vi "Calibrate Camera.vi"(0 "Image In":T1, 5 "Image Dst":T1, 7 "File Path (Image Calibration 1)":path=path "C:/Users/wobot/OneDrive/Desktop/Calibrations/Dots/Cam2.png", 9 "Angle Relative to Horizontal (deg)":sgl, 11 "error in":errorcluster) -> (4 "Image Out":T1, 8 "Execution Time":u32, 15 "error out":errorcluster)   [LabVIEW 2025]
doc: "Creates, edits, and runs vision algorithms using NI Vision Assistant.\n\nWhen you place this Express VI on the block diagram, NI Vision Assistant launches. Create an algorithm using the Vision Assistant processing functions. After you create an algorithm, you can select the controls and indicators that you want to be able to programmatically set in LabVIEW. Double-click the Vision Assistant Express VI to edit the algorithm."
uses:
  <vilib>/vision/Image Controls.llb/IMAQ Image.ctl
  <vilib>/vision/NI_Vision_Development_Module.lvlib
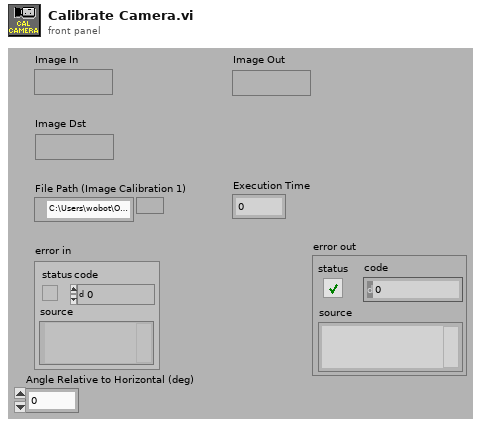
[diagram p1: front panel]
types:
  T1 = typedef "IMAQ Image.ctl" = refnum<image>
  T2 = cluster{"Origin Pixel":cluster{"X":sgl, "Y":sgl}, "Angle Relative to Horizontal (deg)":sgl, "Axis Reference":u32}
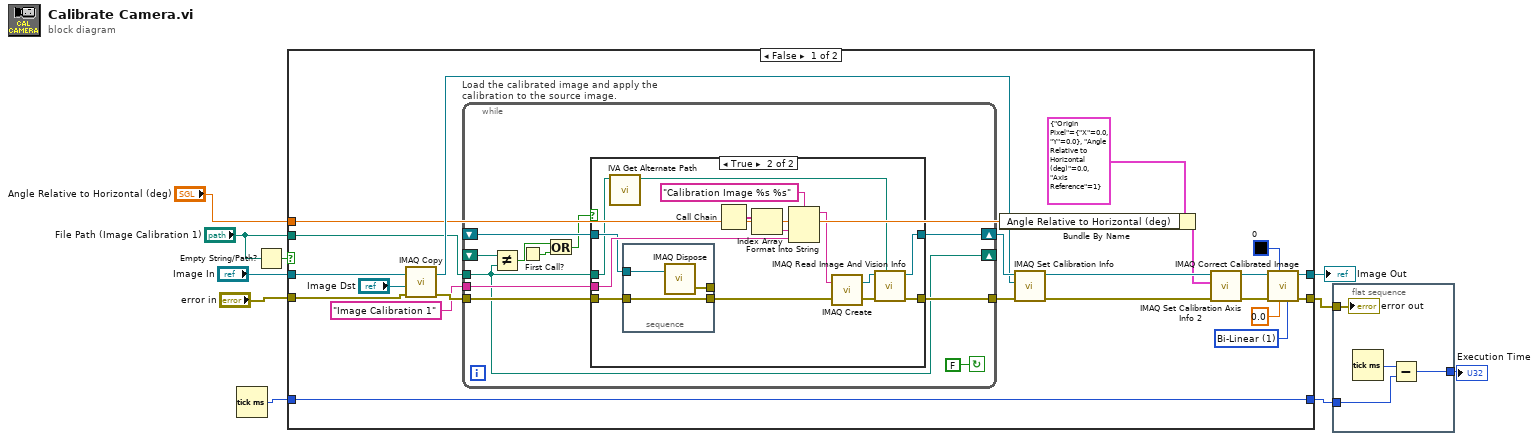
[diagram p0: block diagram]
diagram:
  n1 = Tick Count (ms)() -> (millisecond timer value=w5:u32)
  n2 = Empty String/Path?(string/path="File Path (Image Calibration 1)") -> (empty?=w7:bool)
  n3 = case shown="False" w7 {
    tunnel: "Image In" -> [w31 w64]
    tunnel: [w21 _] -> w4
    tunnel: [w17 w64] -> w9
    tunnel: "File Path (Image Calibration 1)" -> [w16 _]
    tunnel: "error in" -> [w15 _]
    tunnel: w5 -> [w14 w63]
    tunnel: [w14 w63] -> w3
    tunnel: "Angle Relative to Horizontal (deg)" -> [w11 _]
    frame False {
      w22 = u32 1 items=["Zero Order", "Bi-Linear", "Quadratic", "Cubic Spline"] ("Interpolation Type")
      n4 = call "IMAQ Copy"("error in (no error)"=w15, "Image Dst"="Image Dst", "Image Src"=w31) -> ("error out"=w30:errorcluster, "Image Dst Out"=w26:T1)  [unwired: 3 out]
      n5 = while "Load the calibrated image and apply the calibration to the source image." {
        shift-right: [w43] -> w29
        shift-left: _ -> [w42]
        tunnel: [w40] -> w28
        tunnel: w30 -> [w39]
        tunnel: w16 -> [w36]
        tunnel: "Image Calibration 1" ("Step Name") -> [w38]
        shift-right: [w36] -> _
        shift-left: _ -> [w37]
        stop <- FALSE continue-if-true
        n6 = Not Equal?(x=w37, y=w36) -> (x != y?=w34:bool)
        n7 = First Call?() -> (First Call?: T/F=w35:bool)
        n8 = Or(x=w34, y=w35) -> (x .or. y?=w33:bool)
        n9 = case shown="True" w33 {
          tunnel: [w45 w57] -> w43
          tunnel: w42 -> [w45 w49]
          tunnel: [w44 w54] -> w40
          tunnel: w39 -> [w44 w50]
          tunnel: w36 -> [_ w47]
          tunnel: w38 -> [_ w51]
          frame False {
          }
          frame True {
            n10 = call <vilib>:"IVA Get Alternate Path.vi"("Path In"=w47) -> ("Path Out"=w46:path)  [unwired: 10 out]
            n11 = stacked-sequence {
              tunnel: w50 -> [w61]
              tunnel: w49 -> [w62]
              tunnel: [w61] -> w48
              tunnel: [w60] -> _
              frame #0 {
                n12 = call "IMAQ Dispose"("Image"=w62) -> ("error out"=w60:errorcluster)  [unwired: 2 in, 3 out]
              }
            }
            n13 = Call Chain() -> (call chain=w53:string[])
            n14 = Index Array(array=w53) -> (element=w52:string)  [unwired: 1 in]
            n15 = Format Into String(format string="Calibration Image %s %s" ("Image Name"), w52, w51) -> (resulting string=w59:string)  [unwired: 2 in, 1 out]
            n16 = call "IMAQ Create"("Image Name"=w59, "error in (no error)"=w48) -> ("New Image"=w56:T1, "error out"=w55:errorcluster)  [unwired: 2 in, 1 out]
            n17 = call "IMAQ Read Image And Vision Info"("File Path"=w46, "error in (no error)"=w55, "Image"=w56) -> ("error out"=w54:errorcluster, "Image Out"=w57:T1)  [unwired: 1 in, 6 out]
          }
        }
      }
      n18 = Bundle By Name(cluster=T2 {"Origin Pixel"={"X"=0.0, "Y"=0.0}, "Angle Relative to Horizontal (deg)"=0.0, "Axis Reference"=1} ("Calibration Axis Info"), "Angle Relative to Horizontal (deg)"=w11) -> (w12:T2)
      n19 = call "IMAQ Set Calibration Info"("error in (no error)"=w28, "Image Dst"=w26, "Image Src"=w29) -> ("error out"=w27:errorcluster, "Calibrated Image"=w23:T1)  [unwired: 1 in, 6 out]
      n20 = call-poly "IMAQ Set Calibration Axis Info 2"("error in (no error)"=w27, "Calibration Axis Info"=w12, "Calibration Template Image In"=w23) -> ("error out"=w24:errorcluster, "Calibration Template Image Out"=w20:T1)  [unwired: 7 out]
      n21 = call "IMAQ Correct Calibrated Image"("Interpolation Type"=w22, "Replace Value"=sgl 0.0, "Color Replace Value"=u32 0, "error in (no error)"=w24, "Image Src"=w20) -> ("error out"=w21:errorcluster, "Corrected Image"=w17:T1)  [unwired: 2 in, 3 out]
    }
    frame True {
    }
  }
  "Image Out" <- w9
  n22 = flat-sequence {
    tunnel: w4 -> [w65]
    tunnel: w3 -> [w67]
    tunnel: [w66] -> w2
    frame #0 {
      n23 = Tick Count (ms)() -> (millisecond timer value=w68:u32)
      n24 = Subtract(x=w68, y=w67) -> (x-y=w66:u32)
      "error out" <- w65
    }
  }
  "Execution Time" <- w2
